vi "Anomaly Debug (RT).vi"() -> ()   [LabVIEW 2019]
uses:
  <vilib>/Utility/file.llb/Read From Spreadsheet File (DBL).vi
  <vilib>/ptbypt/NI_PtbyPt.lvlib
panel:
  out "subarray":dbl[](array[numeric])
  out "Array 2":i32[](array[numeric])
  out "Waveform Graph":dbl[](graph)
  out "Array":i32[][](array[numeric])
  in  "Points to Avg":i32=20
  in  "Step Threshold":fxp<+/-,28,17>=0.02978515625
  in  "Enable Anomalies":bool[](array[boolean])=[FALSE, FALSE, FALSE, FALSE, FALSE, FALSE, FALSE, FALSE, FALSE, FALSE]
  in  "Anomaly Resets":bool[](array[boolean])=[FALSE, FALSE, FALSE, FALSE, FALSE, FALSE, FALSE, FALSE, FALSE, FALSE]
  out "Steps":u32[](array[numeric])
  in  "Normal Steps":u32=98
  out "Anomalies/Cycle":i32[](array[numeric])
  out "Anomalies (Total)":i32[](array[numeric])
  out "Anomalies (Last Cycle)":i32[](array[numeric])
  in  "Anomaly Threshold":fxp<+/-,28,17>=0.02978515625
  out "Anomaly Array":fxp<+/-,29,18>[](array[numeric])
  in  "Cycle Threshold":fxp<+/-,28,17>=1.2001953125
  in  "Enable Cycles":bool[](array[boolean])=[FALSE, FALSE, FALSE, FALSE, FALSE, FALSE, FALSE, FALSE, FALSE, FALSE]
  in  "Cycle Resets":bool[](array[boolean])=[FALSE, FALSE, FALSE, FALSE, FALSE, FALSE, FALSE, FALSE, FALSE, FALSE]
  out "Total Cycles":u32[](array[numeric])
  out "Cycles":u32[](array[numeric])
  out "Cycle Starts":bool[](array[boolean])
  # "position"
  # "error count"
  # "row"
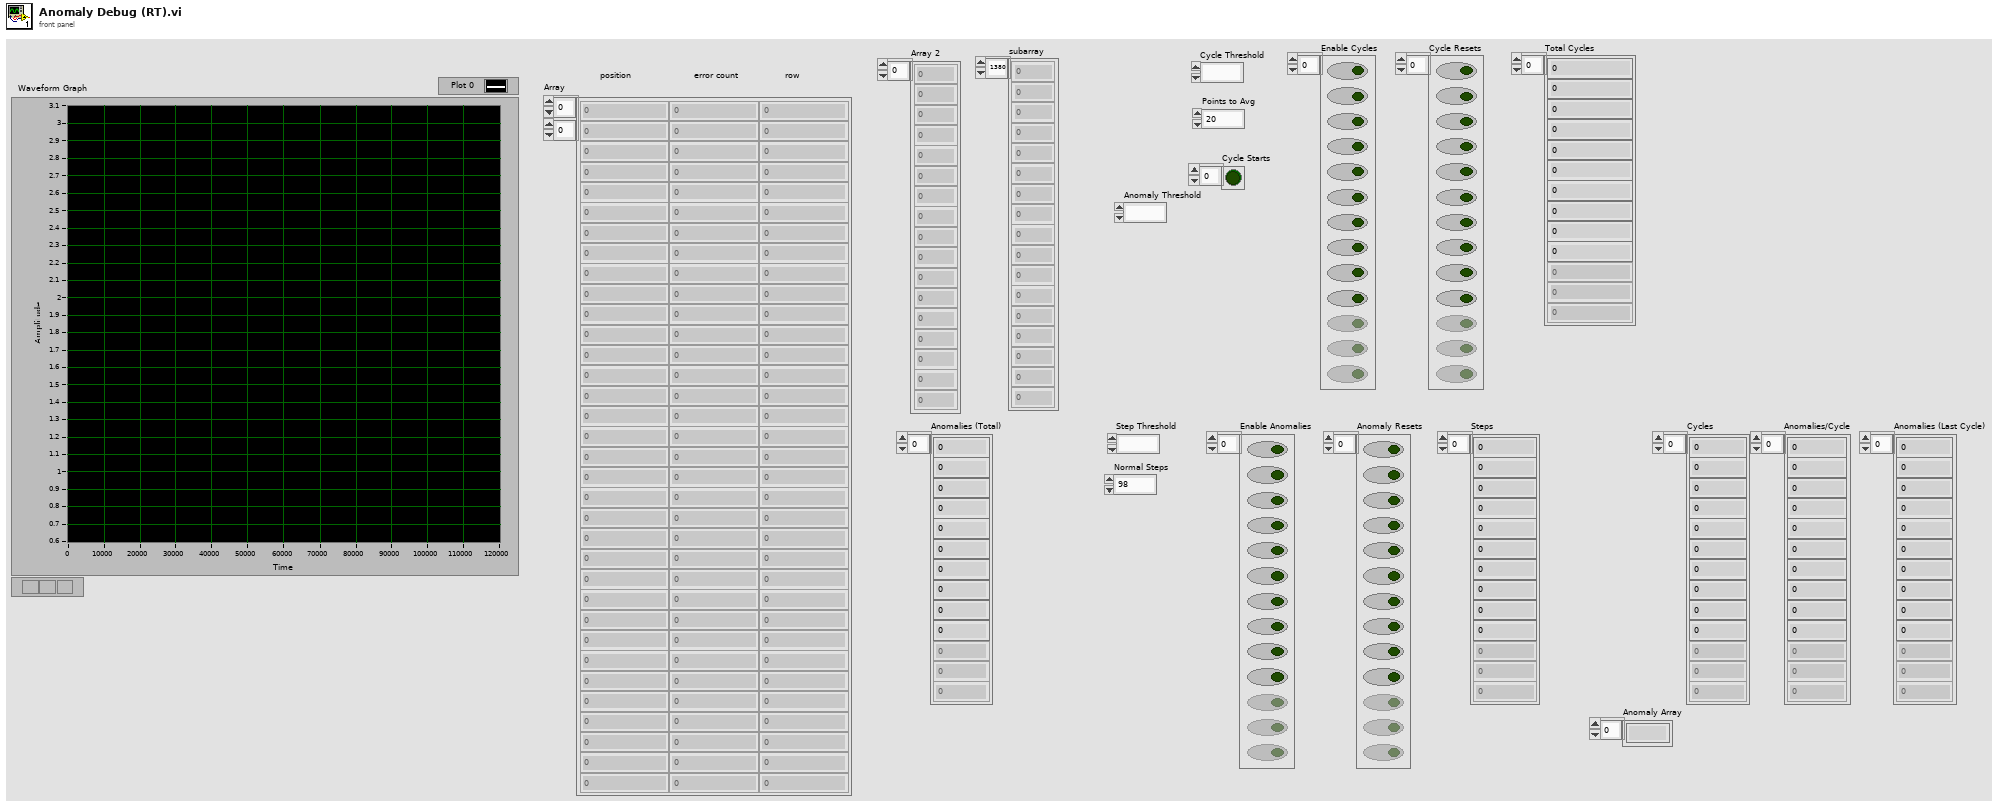
[diagram p1: front panel]
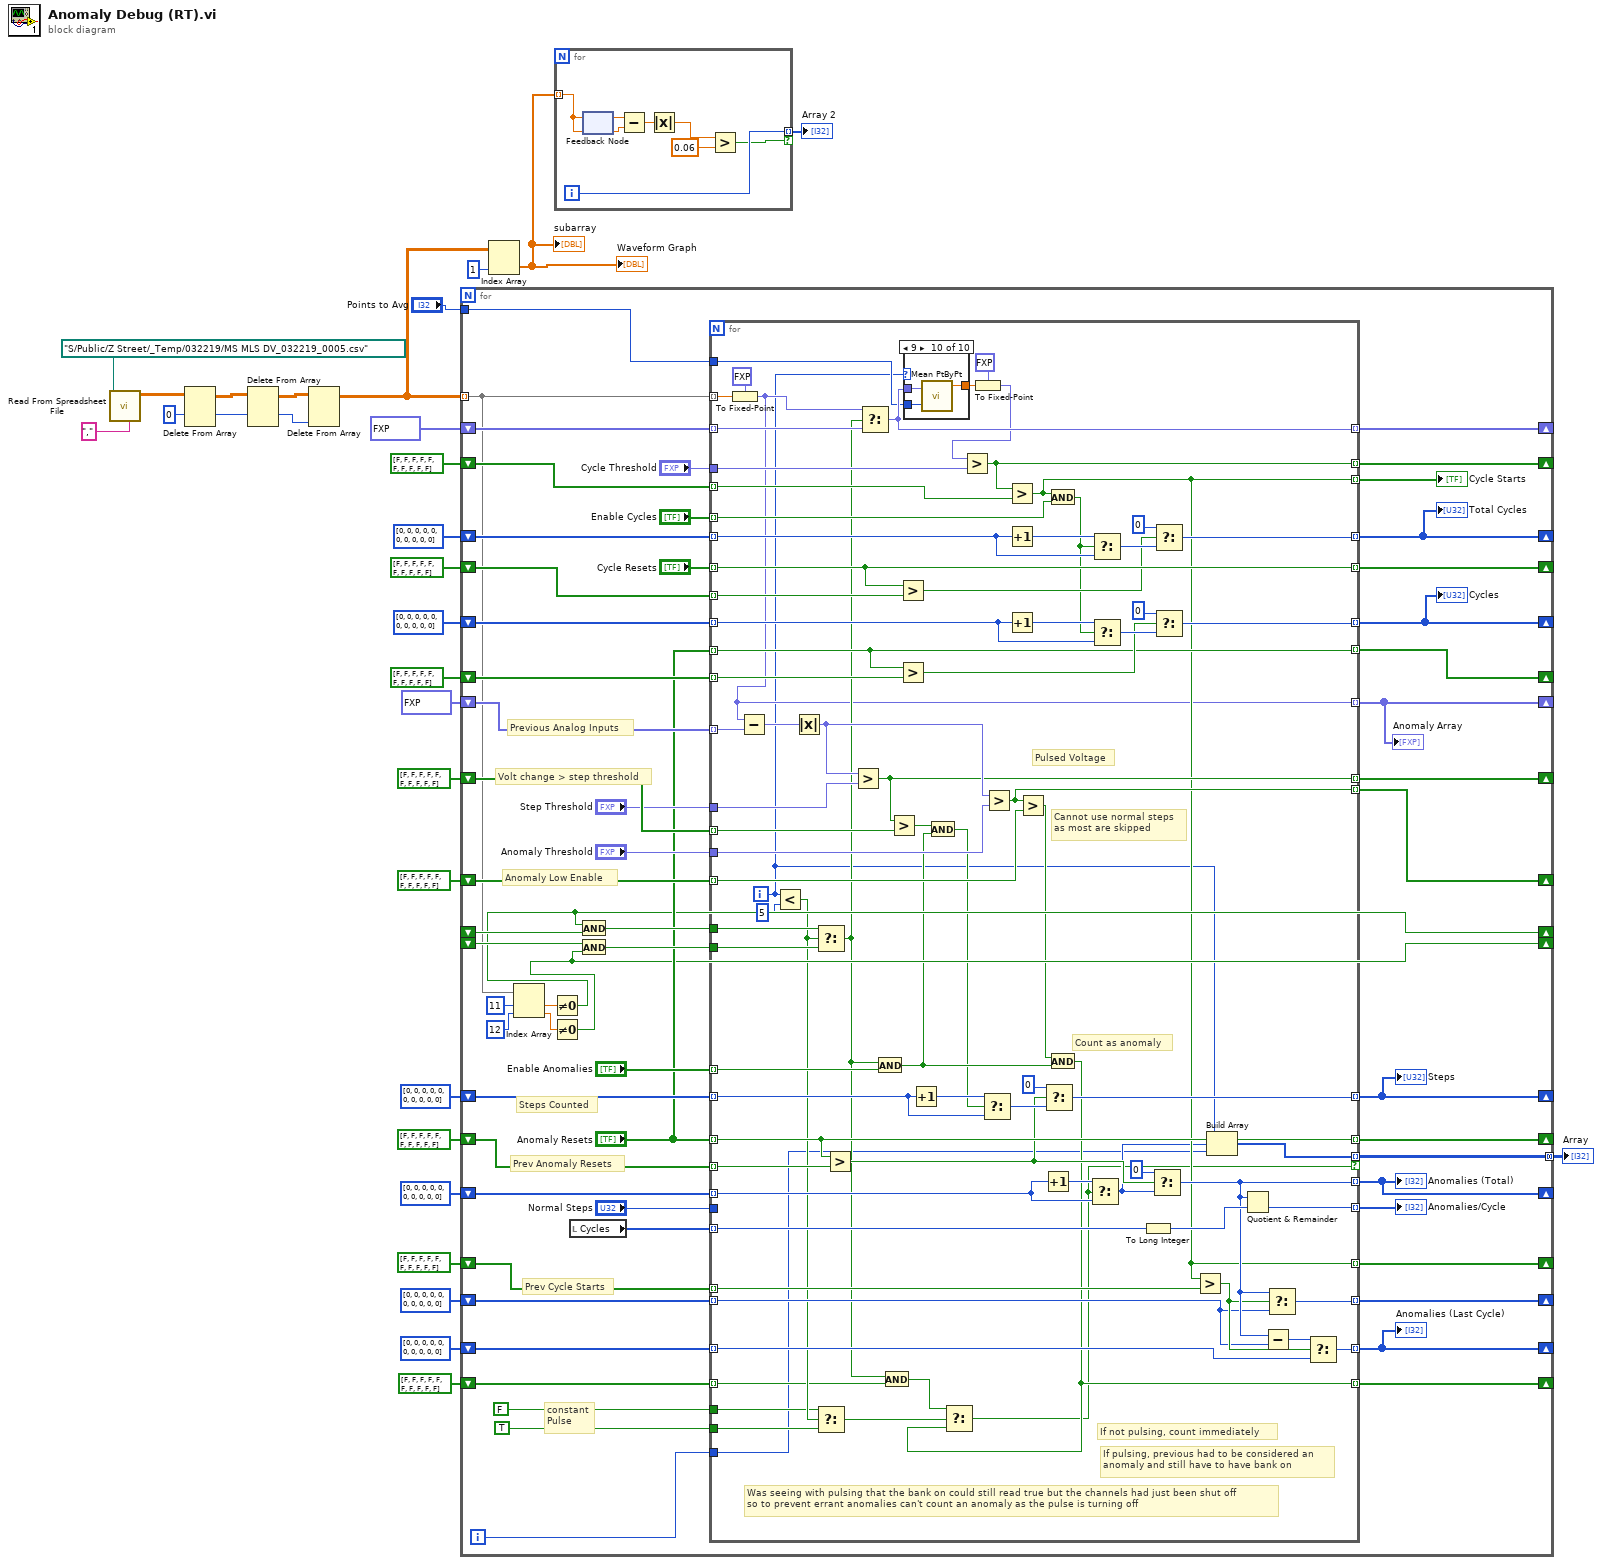
[diagram p0: block diagram]
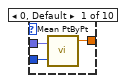
[diagram p2: hidden frame]
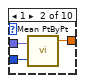
[diagram p3: hidden frame]
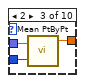
[diagram p4: hidden frame]
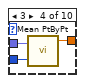
[diagram p5: hidden frame]
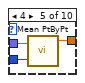
[diagram p6: hidden frame]
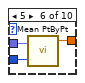
[diagram p7: hidden frame]
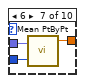
[diagram p8: hidden frame]
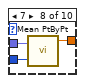
[diagram p9: hidden frame]
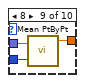
[diagram p10: hidden frame]
diagram:
  w11 = 0 ("index (row)")
  n1 = call-poly <vilib>:"Read From Spreadsheet File.vi"("delimiter (\\t)"="," ("delimiter (\\t)"), "file path (dialog if empty)"=path "S:/Public/Z Street/_Temp/032219/MS MLS DV_032219_0005.csv") -> ("all rows"=w12:dbl[][])  [unwired: 5 in, 4 out]
  n2 = Delete From Array(array=w12, index (row)=w11) -> (array with subset deleted=w10:dbl[][])  [unwired: 2 in, 1 out]
  n3 = Delete From Array(array=w10, index (row)=w11) -> (array with subset deleted=w9:dbl[][])  [unwired: 2 in, 1 out]
  n4 = Delete From Array(array=w9, index (col)=w11) -> (array with subset deleted=w5:dbl[][])  [unwired: 2 in, 1 out]
  n5 = for {
    shift-right: [w82] -> _
    shift-left: bool[] [FALSE, FALSE, FALSE, FALSE, FALSE, FALSE, FALSE, FALSE, FALSE, FALSE] -> [w81]
    shift-right: [w79] -> _
    shift-left: u32[] [0, 0, 0, 0, 0, 0, 0, 0, 0, 0] -> [w78]
    shift-right: [w77] -> _
    shift-left: bool[] [FALSE, FALSE, FALSE, FALSE, FALSE, FALSE, FALSE, FALSE, FALSE, FALSE] -> [w75]
    shift-right: [w84] -> _
    shift-left: fxp<+/-,28,17>[] [0.0, 0.0, 0.0, 0.0, 0.0, 0.0, 0.0, 0.0, 0.0, 0.0] -> [w83]
    shift-right: [w73] -> _
    shift-left: bool[] [FALSE, FALSE, FALSE, FALSE, FALSE, FALSE, FALSE, FALSE, FALSE, FALSE] -> [w72]
    shift-right: [w71] -> _
    shift-left: i32[] [0, 0, 0, 0, 0, 0, 0, 0, 0, 0] -> [w69]
    shift-right: [w70] -> _
    shift-left: i32[] [0, 0, 0, 0, 0, 0, 0, 0, 0, 0] -> [w68]
    shift-right: [w34] -> _
    shift-right: [w33] -> _
    shift-right: [w67] -> _
    shift-left: i32[] [0, 0, 0, 0, 0, 0, 0, 0, 0, 0] -> [w66]
    shift-right: [w63] -> _
    shift-left: bool[] [FALSE, FALSE, FALSE, FALSE, FALSE, FALSE, FALSE, FALSE, FALSE, FALSE] -> [w64]
    shift-left: _ -> [w61]
    shift-left: _ -> [w62]
    tunnel: "Points to Avg" -> [w42]
    shift-right: [w43] -> _
    shift-left: fxp<+/-,28,17>[] [0.0, 0.0, 0.0, 0.0, 0.0, 0.0, 0.0, 0.0, 0.0, 0.0] ("Analog Inputs") -> [w44]
    shift-right: [w45] -> _
    shift-left: bool[] [FALSE, FALSE, FALSE, FALSE, FALSE, FALSE, FALSE, FALSE, FALSE, FALSE] -> [w47]
    shift-right: [w50] -> _
    shift-left: u32[] [0, 0, 0, 0, 0, 0, 0, 0, 0, 0] -> [w51]
    shift-right: [w52] -> _
    shift-left: bool[] [FALSE, FALSE, FALSE, FALSE, FALSE, FALSE, FALSE, FALSE, FALSE, FALSE] -> [w54]
    shift-right: [w56] -> _
    shift-left: u32[] [0, 0, 0, 0, 0, 0, 0, 0, 0, 0] -> [w57]
    shift-right: [w55] -> _
    shift-left: bool[] [FALSE, FALSE, FALSE, FALSE, FALSE, FALSE, FALSE, FALSE, FALSE, FALSE] -> [w59]
    shift-right: [w41] -> _
    shift-left: bool[] [FALSE, FALSE, FALSE, FALSE, FALSE, FALSE, FALSE, FALSE, FALSE, FALSE] -> [w40]
    tunnel: w5 -> [w39] mode=indexing
    tunnel: [w31] -> w8 mode=concatenating
    i -> [w32]
    # "constant\nPulse"
    # "Anomaly Low Enable"
    # "Prev Cycle Starts"
    # "Prev Anomaly Resets"
    # "Steps Counted"
    # "Volt change > step threshold"
    # "Previous Analog Inputs"
    n6 = Index Array(array=w39, index #1=11 ("index"), index #2=12 ("index")) -> (element #1=w36:dbl, element #2=w35:dbl)
    n7 = Not Equal To 0?(x=w36) -> (x != 0?=w34:bool)
    n8 = Not Equal To 0?(x=w35) -> (x != 0?=w33:bool)
    n9 = local read "Cycles"() -> (w74:u32[])
    n10 = And(x=w34, y=w62) -> (x .and. y?=w86:bool)
    n11 = And(x=w61, y=w33) -> (x .and. y?=w85:bool)
    n12 = for {
      tunnel: [w134] -> w82 mode=indexing
      tunnel: w81 -> [w148] mode=indexing
      tunnel: w78 -> [w142] mode=indexing
      tunnel: [w141] -> w79 mode=indexing
      tunnel: "Step Threshold" -> [w135]
      tunnel: "Enable Anomalies" -> [w111] mode=indexing
      tunnel: "Anomaly Resets" -> [w150] mode=indexing
      tunnel: [w150] -> w77 mode=indexing
      tunnel: w75 -> [w151] mode=indexing
      tunnel: [w93] -> w84 mode=indexing
      tunnel: w83 -> [w165] mode=indexing
      tunnel: "Normal Steps" -> [_]
      tunnel: w74 -> [w157] mode=indexing
      tunnel: [w156] -> w76 mode=indexing
      tunnel: [w158] -> w67 mode=indexing
      tunnel: [w109] -> w73 mode=indexing
      tunnel: w72 -> [w153] mode=indexing
      tunnel: [w155] -> w71 mode=indexing
      tunnel: w69 -> [w140] mode=indexing
      tunnel: [w154] -> w70 mode=indexing
      tunnel: w68 -> [w139] mode=indexing
      tunnel: w86 -> [w170]
      tunnel: w85 -> [w169]
      tunnel: w66 -> [w167] mode=indexing
      tunnel: "Anomaly Threshold" -> [w163]
      tunnel: w64 -> [w162] mode=indexing
      tunnel: [w161] -> w63 mode=indexing
      tunnel: w59 -> [w133] mode=indexing
      tunnel: "Anomaly Resets" -> [w126] mode=indexing
      tunnel: w57 -> [w129] mode=indexing
      tunnel: [w128] -> w56 mode=indexing
      tunnel: [w126] -> w55 mode=indexing
      tunnel: w54 -> [w125] mode=indexing
      tunnel: "Cycle Resets" -> [w124] mode=indexing
      tunnel: [w124] -> w52 mode=indexing
      tunnel: w51 -> [w119] mode=indexing
      tunnel: [w118] -> w50 mode=indexing
      tunnel: "Enable Cycles" -> [w117] mode=indexing
      tunnel: "Cycle Threshold" -> [w114]
      tunnel: w47 -> [w115] mode=indexing
      tunnel: [w109] -> w46 mode=indexing
      tunnel: [w113] -> w45 mode=indexing
      tunnel: w44 -> [w112] mode=indexing
      tunnel: [w100] -> w43 mode=indexing
      tunnel: w42 -> [w99]
      tunnel: FALSE -> [w107]
      tunnel: TRUE -> [w106]
      tunnel: [w104] -> w41 mode=indexing
      tunnel: w40 -> [w102] mode=indexing
      tunnel: w39 -> [w95] mode=indexing
      tunnel: w32 -> [w91]
      tunnel: [w90] -> w31 mode=indexing if=w89
      i -> [w88]
      # "If pulsing, previous had to be considered an\nanomaly and still have to have bank on"
      # "If not pulsing, count immediately"
      # "Count as anomaly"
      # "Was seeing with pulsing that the bank on could still read true but the channels had just been shut off\nso to prevent errant anomalies can't count an anomaly as the pulse is turning off"
      # "Cannot use normal steps\nas most are skipped"
      # "Pulsed Voltage"
      n13 = To Fixed-Point(fixed-point type=fxp<+/-,28,17> 0.0 ("AI0"), number=w95) -> (fixed-point=w93:fxp<+/-,28,17>)
      n14 = Subtract(x=w93, y=w165) -> (x-y=w166:fxp<+/-,29,18>)
      n15 = Less?(x=w88, y=5) -> (x < y?=w108:bool)
      n16 = Absolute Value(x=w166) -> (abs(x)=w164:fxp<+,28,17>)
      n17 = Select(t=w170, s=w108, f=w169) -> (s? t:f=w103:bool)
      n18 = Select(t=w107, s=w108, f=w106) -> (s? t:f=w105:bool)
      n19 = Greater?(x=w150, y=w151) -> (0:w143:bool)
      n20 = Greater?(x=w164, y=w135) -> (0:w134:bool)
      n21 = Select(t=w93, s=w103, f=w112) -> (s? t:f=w100:fxp<+/-,28,17>)
      n22 = And(x=w103, y=w111) -> (x .and. y?=w147:bool)
      n23 = And(x=w103, y=w102) -> (x .and. y?=w101:bool)
      n24 = Greater?(x=w134, y=w148) -> (0:w149:bool)
      n25 = Greater?(x=w124, y=w125) -> (0:w120:bool)
      n26 = Greater?(x=w126, y=w133) -> (0:w127:bool)
      n27 = case shown="9" w88 {
        tunnel: w100 -> [w173 w176 w179 w182 w185 w188 w191 w194 w197 w200]
        tunnel: w99 -> [w172 w175 w178 w181 w184 w187 w190 w193 w196 w199]
        tunnel: [w171 w174 w177 w180 w183 w186 w189 w192 w195 w198] -> w98
        frame 0, Default {
          n28 = call <vilib>:"Mean PtByPt.vi"("x"=w173, "sample length"=w172) -> ("mean"=w171:dbl)  [unwired: 2 in, 1 out]
        }
        frame 1 {
          n29 = call <vilib>:"Mean PtByPt.vi"("x"=w176, "sample length"=w175) -> ("mean"=w174:dbl)  [unwired: 2 in, 1 out]
        }
        frame 2 {
          n30 = call <vilib>:"Mean PtByPt.vi"("x"=w179, "sample length"=w178) -> ("mean"=w177:dbl)  [unwired: 2 in, 1 out]
        }
        frame 3 {
          n31 = call <vilib>:"Mean PtByPt.vi"("x"=w182, "sample length"=w181) -> ("mean"=w180:dbl)  [unwired: 2 in, 1 out]
        }
        frame 4 {
          n32 = call <vilib>:"Mean PtByPt.vi"("x"=w185, "sample length"=w184) -> ("mean"=w183:dbl)  [unwired: 2 in, 1 out]
        }
        frame 5 {
          n33 = call <vilib>:"Mean PtByPt.vi"("x"=w188, "sample length"=w187) -> ("mean"=w186:dbl)  [unwired: 2 in, 1 out]
        }
        frame 6 {
          n34 = call <vilib>:"Mean PtByPt.vi"("x"=w191, "sample length"=w190) -> ("mean"=w189:dbl)  [unwired: 2 in, 1 out]
        }
        frame 7 {
          n35 = call <vilib>:"Mean PtByPt.vi"("x"=w194, "sample length"=w193) -> ("mean"=w192:dbl)  [unwired: 2 in, 1 out]
        }
        frame 8 {
          n36 = call <vilib>:"Mean PtByPt.vi"("x"=w197, "sample length"=w196) -> ("mean"=w195:dbl)  [unwired: 2 in, 1 out]
        }
        frame 9 {
          n37 = call <vilib>:"Mean PtByPt.vi"("x"=w200, "sample length"=w199) -> ("mean"=w198:dbl)  [unwired: 2 in, 1 out]
        }
      }
      n38 = Increment(x=w142) -> (x+1=w144:u32)
      n39 = And(x=w149, y=w147) -> (x .and. y?=w110:bool)
      n40 = To Fixed-Point(fixed-point type=fxp<+/-,28,17> 0.0 ("Averaged Data"), number=w98) -> (fixed-point=w96:fxp<+/-,28,17>)
      n41 = Greater?(x=w96, y=w114) -> (0:w113:bool)
      n42 = Select(t=w144, s=w110, f=w142) -> (s? t:f=w145:u32)
      n43 = Greater?(x=w164, y=w163) -> (0:w161:bool)
      n44 = Greater?(x=w113, y=w115) -> (0:w109:bool)
      n45 = Increment(x=w119) -> (x+1=w121:u32)
      n46 = Increment(x=w129) -> (x+1=w132:u32)
      n47 = Greater?(x=w161, y=w162) -> (0:w136:bool)
      n48 = Increment(x=w167) -> (x+1=w137:i32)
      n49 = Select(t=u32 0, s=w143, f=w145) -> (s? t:f=w141:u32)
      n50 = And(x=w109, y=w117) -> (x .and. y?=w116:bool)
      n51 = And(x=w136, y=w147) -> (x .and. y?=w104:bool)
      n52 = Select(t=w101, s=w105, f=w104) -> (s? t:f=w89:bool)
      n53 = Select(t=w137, s=w89, f=w167) -> (s? t:f=w92:i32)
      n54 = Select(t=w121, s=w116, f=w119) -> (s? t:f=w122:u32)
      n55 = Select(t=w132, s=w116, f=w129) -> (s? t:f=w131:u32)
      n56 = To Long Integer(number=w157) -> (32bit integer=w159:i32)
      n57 = Select(t=0, s=w143, f=w92) -> (s? t:f=w158:i32)
      n58 = Select(t=u32 0, s=w120, f=w122) -> (s? t:f=w118:u32)
      n59 = Select(t=u32 0, s=w127, f=w131) -> (s? t:f=w128:u32)
      n60 = Greater?(x=w109, y=w153) -> (0:w152:bool)
      n61 = Build Array(w88, w92, w91) -> (w90:i32[])
      n62 = Quotient & Remainder(x=w158, y=w159) -> (floor(x/y)=w156:i32)  [unwired: 1 out]
      n63 = Subtract(x=w158, y=w140) -> (x-y=w160:i32)
      n64 = Select(t=w158, s=w152, f=w140) -> (s? t:f=w155:i32)
      n65 = Select(t=w160, s=w152, f=w139) -> (s? t:f=w154:i32)
    }
    "Steps" <- w79
    "Anomalies/Cycle" <- w76
    "Anomalies (Total)" <- w67
    "Anomalies (Last Cycle)" <- w70
    "Anomaly Array" <- w84
    "Total Cycles" <- w50
    "Cycles" <- w56
    "Cycle Starts" <- w46
  }
  "Array" <- w8
  n66 = Index Array(array=w5, index (col)=1 ("disabled index (col)")) -> (element=w3:dbl[])  [unwired: 1 in]
  "Waveform Graph" <- w3
  "subarray" <- w3
  n67 = for {
    tunnel: w3 -> [w206] mode=indexing
    tunnel: [w202] -> w2 mode=indexing if=w201
    i -> [w202]
    n68 = feedback-in #1(w206) -> ()
    n69 = feedback #1(w206) -> (w207:dbl)
    n70 = Subtract(x=w207, y=w206) -> (x-y=w205:dbl)
    n71 = Absolute Value(x=w205) -> (abs(x)=w204:dbl)
    n72 = Greater?(x=w204, y=0.06) -> (0:w201:bool)
  }
  "Array 2" <- w2
